vi "Write Array Element.vi"(5 "element":refnum<class "Control.lvclass">, 9 "Array in":refnum<class "Array.lvclass">) -> (3 "Array out":refnum<class "Array.lvclass">)   [LabVIEW 2014, in "Array.lvclass"]
uses:
  Array.lvclass
  Control/Control.lvclass
  Array.lvclass/Array.ctl
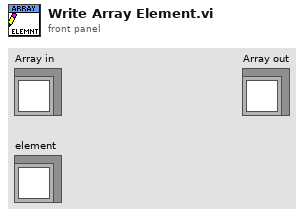
[diagram p1: front panel]
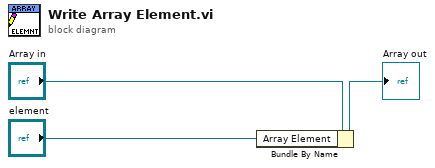
[diagram p0: block diagram]
diagram:
  n1 = Bundle By Name(cluster="Array in", "Array Element"="element") -> (→"Array out":refnum<class "Array.lvclass">)
